vi "NewProductB.vi"(8 "error in (no error)":errorcluster) -> (0 "error out":errorcluster, 3 "ProductB":refnum<class "ProductB.lvclass">)   [LabVIEW 2020, in "FactoryMethod.lvlib" / "FactoryMethodLazyEvaluation.lvlib" / "ProductB.lvclass"]
uses:
  ProductB.lvclass
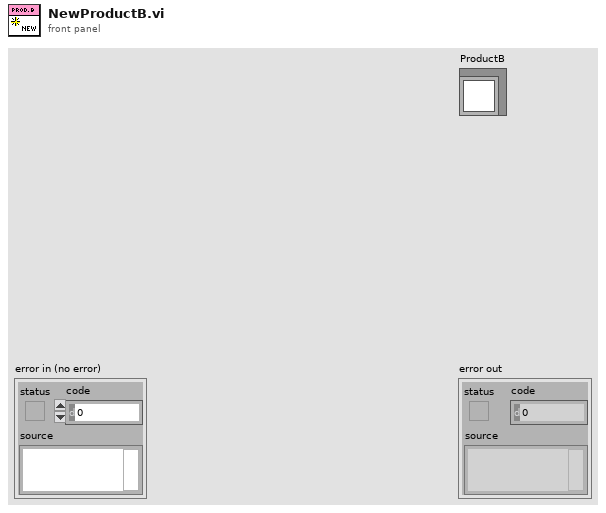
[diagram p1: front panel]
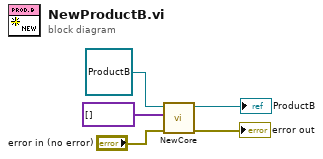
[diagram p0: block diagram]
diagram:
  n1 = call-dynamic "NewCore.vi"("error in (no error)"="error in (no error)", "ParamsArray"=variant[] [], "ProductB"=refnum<class "ProductB.lvclass"> refnum ("ConcreteProductA in")) -> ("error out"=→"error out":errorcluster, "ProductB"=→"ProductB":refnum<class "ProductB.lvclass">)  [unwired: 7 in]
